vi "Set Tx Generic Frame Header List.vi"(8 "error in":errorcluster, 10 "Frame Headers":T1[](array[typedef]) {"Parameters"."Parameter"."encoding" items=["BNR", "BCD", "Discrete"]; "Frame header"."SequenceNumberOffset" items=["FDX_TX_FRAME_SEQ_OFFS_AUTO"=65535]; "Frame header"."SequenceNumberInit" items=["FDX_TX_FRAME_SEQ_INIT_AUTO"=65535, "FDX_TX_FRAME_SEQ_OFF"=65533]; "Frame header"."PhysErrorInjection" items=["FDX_TX_FRAME_ERR_OFF", "FDX_TX_FRAME_ERR_CRC", "FDX_TX_FRAME_ERR_ALI", "FDX_TX_FRAME_ERR_PRE", "FDX_TX_FRAME_ERR_PHY"]; "Frame header"."PayloadGenerationMode" items=["FDX_TX_FRAME_PGM_USER", "FDX_TX_FRAME_PGM_IP_PART", "FDX_TX_FRAME_PGM_IP_PART_TT", "FDX_TX_FRAME_PGM_IP_FULL", "FDX_TX_FRAME_PGM_IP_FULL_TT"]; "Frame header"."PayloadBufferMode" items=["FDX_TX_FRAME_PBM_STD", "FDX_TX_FRAME_PBM_MAC", "FDX_TX_FRAME_PBM_UDP", "FDX_TX_FRAME_PBM_FULL"]; "Frame header"."NetSelect" items=["FDX_TX_FRAME_DLY_A"=0, "FDX_TX_FRAME_DLY_B"=1, "FDX_TX_FRAME_BOTH "=3, "FDX_TX_FRAME_ONLY_A"=4, "FDX_TX_FRAME_ONLY_B "=5]; "Frame header"."FrameStartMode" items=["FDX_TX_FRAME_START_IFG", "FDX_TX_FRAME_START_PGWT", "FDX_TX_FRAME_START_TRG", "FDX_TX_FRAME_START_TRG_D"]}, 11 "custom device ref in":T7 format="%.0x") -> (0 "error out":errorcluster, 3 "custom device ref out":T7 format="%.0x")   [LabVIEW 2020, in "AIM ARINC 664 Scripting.lvlib"]
uses:
  AIM ARINC 664 Scripting.lvlib
  <vilib>/NI VeriStand/Custom Device API/Custom Device API.lvlib
  Constants.vi
  Program Files/National Instruments/LabVIEW 2025/instr.lib/AIM GmbH/_AIM 664/_controls/queue_header_generic.ctl
  Program Files/National Instruments/LabVIEW 2025/instr.lib/AIM GmbH/_AIM 664/AIM664LV.lvlib
  <vilib>/NI VeriStand/Custom Device API/Custom Device Channel Type.ctl
  <vilib>/NI VeriStand/Custom Device API/Custom Device Channel.ctl
  <vilib>/NI VeriStand/Custom Device API/Set Item Property (String).vi
  Shared/RawFrame_entry.ctl
  <vilib>/NI VeriStand/Custom Device API/Set Item Property (U32 Array).vi
  <vilib>/NI VeriStand/Custom Device API/Get Item Property (U32 Array).vi
  <vilib>/NI VeriStand/Custom Device API/Set Item Property (Variant).vi
  <vilib>/NI VeriStand/Custom Device API/Custom Device Item Ref.ctl
  Import/_typedefs/frame_tx_generic_seqNumberInit.ctl
  Import/AIM ARINC 664 Import.lvlib
  Import/_typedefs/frame_tx_generic_seqNumberOffset.ctl
  Import/_typedefs/frame_tx_generic.ctl
  Import/_typedefs/frame_parameter_definition.ctl
  Import/_typedefs/frame_parameter.ctl
  Shared/Encoding (Arinc664).ctl
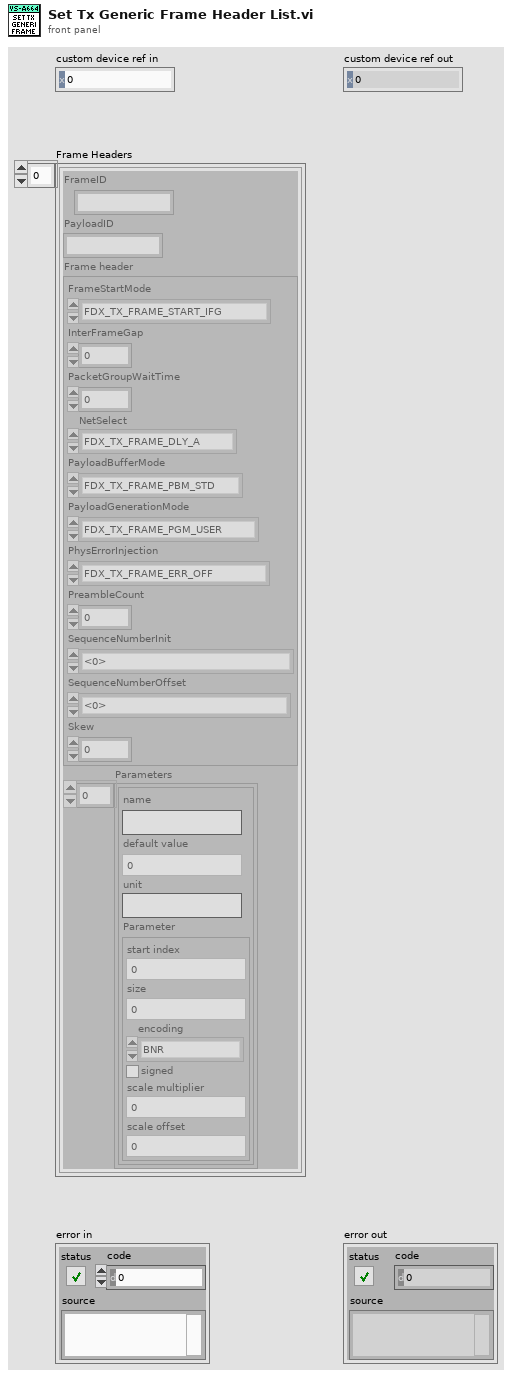
[diagram p1: front panel]
types:
  T1 = typedef "AIM ARINC 664 Import.lvlib/frame_tx_generic.ctl" = cluster{"FrameID":string, "PayloadID":string, "Frame header":cluster{"FrameStartMode":i32, "InterFrameGap":i32, "PacketGroupWaitTime":i32, "NetSelect":u32, "PayloadBufferMode":i32, "PayloadGenerationMode":i32, "PhysErrorInjection":i32, "PreambleCount":i32, "SequenceNumberInit":T2, "SequenceNumberOffset":T3, "Skew":i32}, "Parameters":T4[]}
  T2 = typedef "AIM ARINC 664 Import.lvlib/frame_tx_generic_seqNumberInit.ctl" = i32
  T3 = typedef "AIM ARINC 664 Import.lvlib/frame_tx_generic_seqNumberOffset.ctl" = i32
  T4 = typedef "AIM ARINC 664 Import.lvlib/frame_parameter.ctl" = cluster{"name":string, "default value":dbl, "unit":string, "Parameter":T5}
  T5 = typedef "AIM ARINC 664 Import.lvlib/frame_parameter_definition.ctl" = cluster{"start index":i32, "size":i32, "encoding":T6, "signed":bool, "scale multiplier":dbl, "scale offset":dbl}
  T6 = typedef "Encoding (Arinc664).ctl" = u16
  T7 = typedef "Custom Device API.lvlib/Custom Device Item Ref.ctl" = u64
  T8 = typedef "RawFrame_entry.ctl" = cluster{"HeaderInfo":T9, "PayloadID":string}
  T9 = typedef "AIM664LV.lvlib/queue_header_generic.ctl" = cluster{"InterFrameGap":u32, "PacketGroupWaitTime":u32, "PayloadBufferMode":u8, "PayloadGenerationMode":u8, "PreambleCount":u8, "Skew":u32, "NetSelect":u8, "FrameStartMode":u8, "PhysErrorInjection":u32, "SequenceNumberInit":u16, "SequenceNumberOffset":u16}
  T10 = typedef "Custom Device API.lvlib/Custom Device Channel Type.ctl" = enum16{"Input", "Output"}
  T11 = typedef "Custom Device API.lvlib/Custom Device Channel.ctl" = cluster{"Type":T10, "Units":string, "Default Value":dbl, "Faultable":bool, "Scalable":bool}
  T12 = cluster{"FrameStartMode":i32, "InterFrameGap":i32, "PacketGroupWaitTime":i32, "NetSelect":u32, "PayloadBufferMode":i32, "PayloadGenerationMode":i32, "PhysErrorInjection":i32, "PreambleCount":i32, "SequenceNumberInit":T2, "SequenceNumberOffset":T3, "Skew":i32}
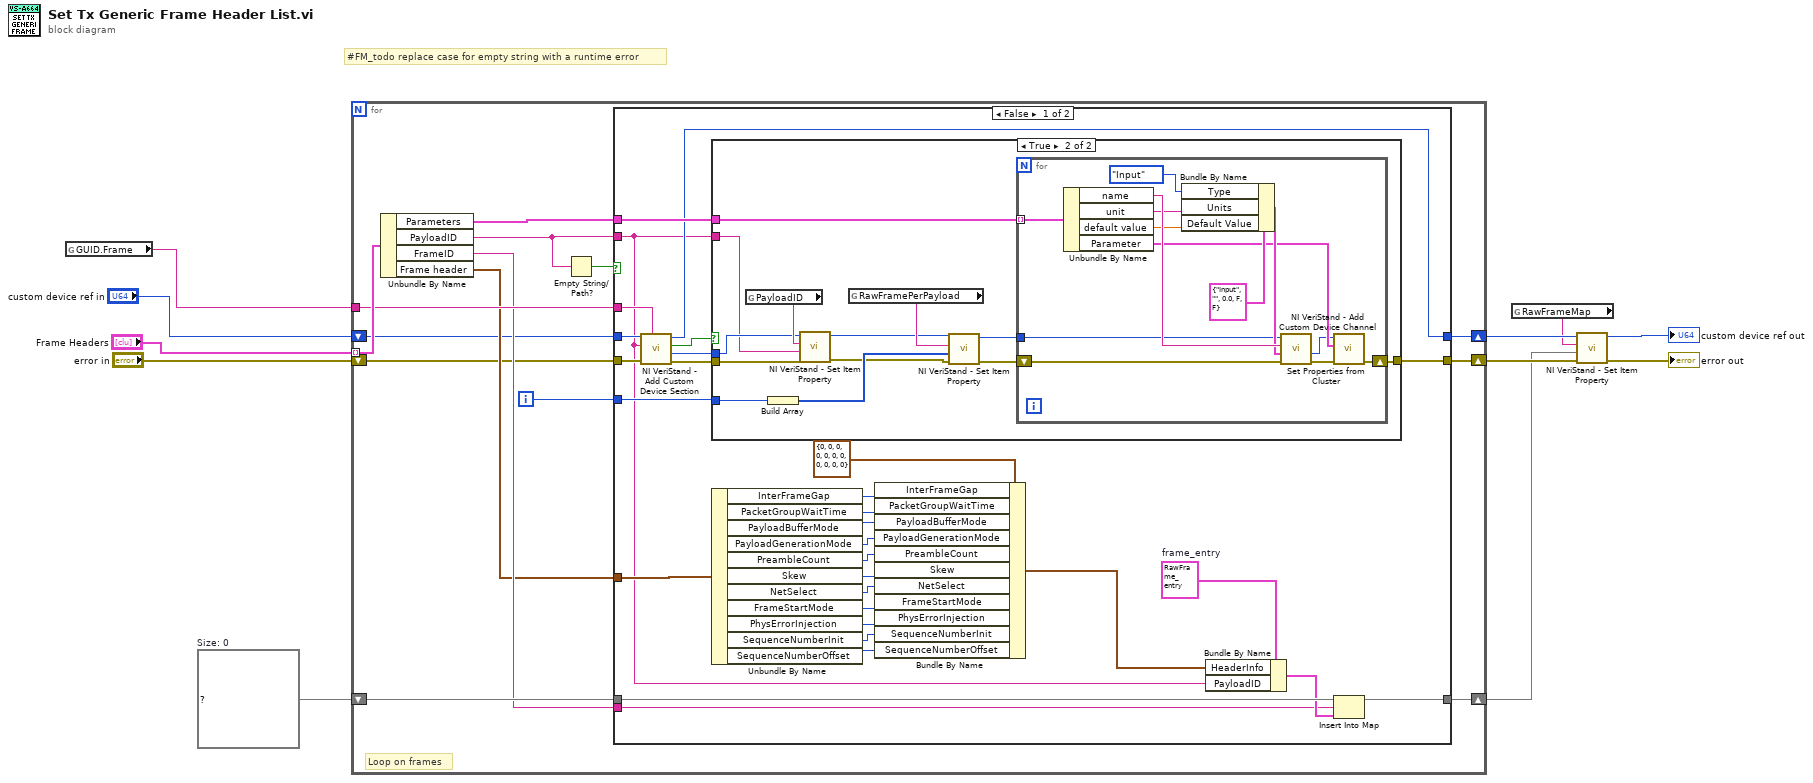
[diagram p0: block diagram]
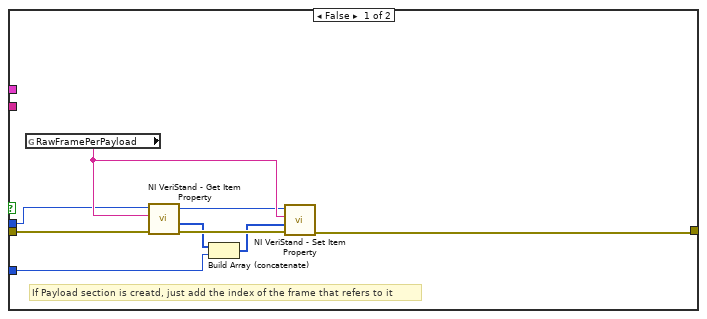
[diagram p2: hidden frame]
diagram:
  w3 = map{string, T8} {}  # Size: 0
  # "#FM_todo replace case for empty string with a runtime error"
  n1 = global read "Constants.vi" "GUID.Frame"() -> (w7:string)
  n2 = for {
    tunnel: "Frame Headers" -> [w25] mode=indexing
    shift-right: [w23] -> w4
    shift-left: "error in" -> [w15]
    shift-right: [w22] -> w5
    shift-left: "custom device ref in" -> [w14]
    tunnel: w7 -> [w21]
    shift-right: [w20] -> w2
    shift-left: w3 -> [w19]
    i -> [w17]
    # "Loop on frames"
    n3 = Unbundle By Name(w25) -> ("Parameters"=w24:T4[], "PayloadID"=w13:string, "FrameID"=w18:string, "Frame header"=w16:T12)
    n4 = Empty String/Path?(string/path=w13) -> (empty?=w12:bool)
    n5 = case shown="False" w12 {
      tunnel: w24 -> [w55 _]
      tunnel: [w54 w92] -> w23
      tunnel: [w50 w91] -> w22
      tunnel: w21 -> [w49 _]
      tunnel: [w47 w93] -> w20
      tunnel: w19 -> [w46 w93]
      tunnel: w18 -> [w44 _]
      tunnel: w17 -> [w43 _]
      tunnel: w16 -> [w40 _]
      tunnel: w15 -> [w28 w92]
      tunnel: w14 -> [w27 w91]
      tunnel: w13 -> [w26 _]
      frame False {
        w48 = T8 {"HeaderInfo"={"InterFrameGap"=0, "PacketGroupWaitTime"=0, "PayloadBufferMode"=0, "PayloadGenerationMode"=0, "PreambleCount"=0, "Skew"=0, "NetSelect"=0, "FrameStartMode"=0, "PhysErrorInjection"=0, "SequenceNumberInit"=65535, "SequenceNumberOffset"=0}, "PayloadID"=""}  # frame_entry
        n6 = call <vilib>:"NI VeriStand - Add Custom Device Section.vi"("GUID (Default Section)"=w49, "error in (no error)"=w28, "Section Name"=w26, "Parent Ref in"=w27) -> ("error out"=w51:errorcluster, "Section Ptr"=w52:T7, "Newly Created?"=w53:bool, "Parent Ref out"=w50:T7)  [unwired: 4 in]
        n7 = case shown="True" w53 {
          tunnel: w55 -> [_ w77]
          tunnel: [w56 w76] -> w54
          tunnel: w51 -> [w64 w74]
          tunnel: w52 -> [w57 w73]
          tunnel: w43 -> [w60 w70]
          tunnel: w26 -> [_ w71]
          frame False {
            # "If Payload section is creatd, just add the index of the frame that refers to it"
            n8 = global read "Constants.vi" "RawFramePerPayload"() -> (w63:string)
            n9 = call-poly <vilib>:"NI VeriStand - Get Item Property.vi"("error in (no error)"=w64, "Property Name"=w63, "Item Ref in"=w57) -> ("error out"=w62:errorcluster, "Value"=w61:u32[], "Item Ref out"=w58:T7)  [unwired: 5 in, 1 out]
            n10 = Build Array (concatenate)(w61, w60) -> (w59:u32[])
            n11 = call-poly <vilib>:"NI VeriStand - Set Item Property.vi"("error in (no error)"=w62, "Value"=w59, "Property Name"=w63, "Item Ref in"=w58) -> ("error out"=w56:errorcluster)  [unwired: 5 in, 2 out]
          }
          frame True {
            n12 = global read "Constants.vi" "PayloadID"() -> (w75:string)
            n13 = Build Array(w70) -> (w69:i32[])
            n14 = call-poly <vilib>:"NI VeriStand - Set Item Property.vi"("error in (no error)"=w74, "Value"=w71, "Property Name"=w75, "Item Ref in"=w73) -> ("error out"=w68:errorcluster, "Item Ref out"=w67:T7)  [unwired: 5 in, 1 out]
            n15 = global read "Constants.vi" "RawFramePerPayload"() -> (w72:string)
            n16 = call-poly <vilib>:"NI VeriStand - Set Item Property.vi"("error in (no error)"=w68, "Value"=w69, "Property Name"=w72, "Item Ref in"=w67) -> ("error out"=w66:errorcluster, "Item Ref out"=w65:T7)  [unwired: 5 in, 1 out]
            n17 = for {
              tunnel: w77 -> [w90] mode=indexing
              shift-right: [w83] -> w76
              shift-left: w66 -> [w79]
              tunnel: w65 -> [w78]
              n18 = Unbundle By Name(w90) -> ("name"=w89:string, "unit"=w86:string, "default value"=w85:dbl, "Parameter"=w82:T5)
              n19 = Bundle By Name(cluster=T11 {"Type"=enum."Input", "Units"="", "Default Value"=0.0, "Faultable"=FALSE, "Scalable"=FALSE} ("Channel"), "Type"=Custom_Device_Channel_Type."Input", "Units"=w86, "Default Value"=w85) -> (w87:T11)
              n20 = call <vilib>:"NI VeriStand - Add Custom Device Channel.vi"("error in (no error)"=w79, "Channel"=w87, "Channel Name"=w89, "Parent Ref in"=w78) -> ("error out"=w84:errorcluster, "Channel Ref"=w81:T7)  [unwired: 4 in, 2 out]
              n21 = call "Set Properties from Cluster.vi"("error in"=w84, "Variant Cluster"=w82, "item ref in"=w81) -> ("error out"=w83:errorcluster)  [unwired: 7 in, 1 out]
            }
          }
        }
        n22 = Unbundle By Name(w40) -> ("InterFrameGap"=w39:i32, "PacketGroupWaitTime"=w38:i32, "PayloadBufferMode"=w37:i32, "PayloadGenerationMode"=w36:i32, "PreambleCount"=w35:i32, "Skew"=w34:i32, "NetSelect"=w33:u32, "FrameStartMode"=w32:i32, "PhysErrorInjection"=w31:i32, "SequenceNumberInit"=w30:T2, "SequenceNumberOffset"=w29:T3)
        n23 = Bundle By Name(cluster=T9 {"InterFrameGap"=0, "PacketGroupWaitTime"=0, "PayloadBufferMode"=0, "PayloadGenerationMode"=0, "PreambleCount"=0, "Skew"=0, "NetSelect"=0, "FrameStartMode"=0, "PhysErrorInjection"=0, "SequenceNumberInit"=0, "SequenceNumberOffset"=0} ("HeaderInfo"), "InterFrameGap"=w39, "PacketGroupWaitTime"=w38, "PayloadBufferMode"=w37, "PayloadGenerationMode"=w36, "PreambleCount"=w35, "Skew"=w34, "NetSelect"=w33, "FrameStartMode"=w32, "PhysErrorInjection"=w31, "SequenceNumberInit"=w30, "SequenceNumberOffset"=w29) -> (w41:T9)
        n24 = Bundle By Name(cluster=w48, "HeaderInfo"=w41, "PayloadID"=w26) -> (w45:T8)
        n25 = Insert Into Map(map in=w46, key=w44, value=w45) -> (map out=w47:map{string, T8})  [unwired: 2 out]
      }
      frame True {
      }
    }
  }
  n26 = global read "Constants.vi" "RawFrameMap"() -> (w1:string)
  n27 = call-poly <vilib>:"NI VeriStand - Set Item Property.vi"("error in (no error)"=w4, "Value"=w2, "Property Name"=w1, "Item Ref in"=w5) -> ("error out"=→"error out":errorcluster, "Item Ref out"=→"custom device ref out":T7)  [unwired: 5 in, 1 out]
